vi "Write send from port.vi"(8 "error in (no error)":errorcluster, 10 "send from port":u16=61556, 11 "TEC configuration in":refnum<class "TEC configuration.lvclass">) -> (0 "error out":errorcluster, 3 "TEC configuration out":refnum<class "TEC configuration.lvclass">)   [LabVIEW 2013, in "TEC configuration.lvclass"]
uses:
  TEC configuration.lvclass
  TEC configuration.lvclass/TEC configuration.ctl
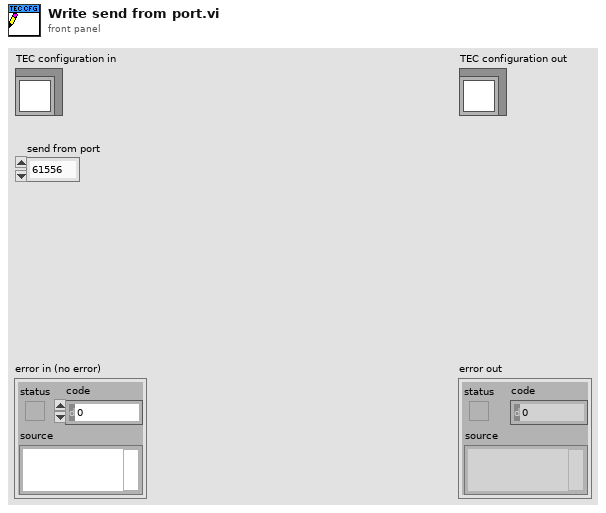
[diagram p1: front panel]
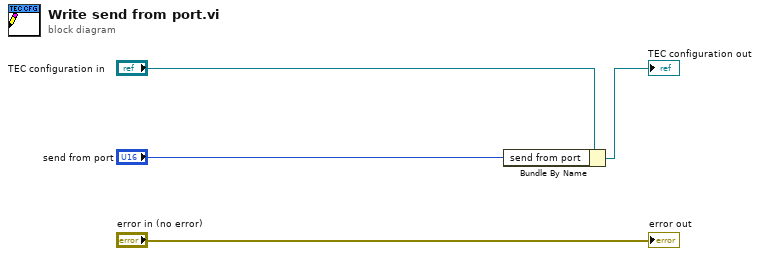
[diagram p0: block diagram]
diagram:
  n1 = Bundle By Name(cluster="TEC configuration in", "send from port"="send from port") -> (→"TEC configuration out":refnum<class "TEC configuration.lvclass">)
  "error out" <- "error in (no error)"
